vi "Event from DBL Ary.vi"(7 "Time Stamp":timestamp, 10 "Array":dbl[](array[numeric]), 11 "VI Refnum":refnum<vi>) -> (2 "Event Data":T1)   [LabVIEW 2023, in "Instruments.lvlib" / "Instruments.lvclass"]
uses:
  Library/Instruments.lvclass
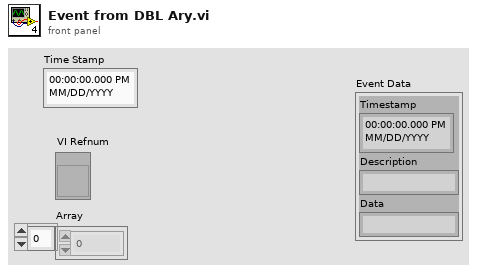
[diagram p1: front panel]
types:
  T1 = cluster{"Timestamp":timestamp, "Description":string, "Data":string}
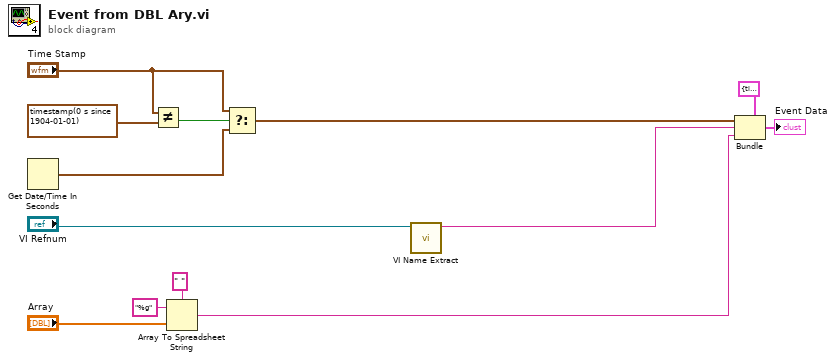
[diagram p0: block diagram]
diagram:
  n1 = Get Date/Time In Seconds() -> (seconds since 1Jan1904=w8:timestamp)
  n2 = Not Equal?(x="Time Stamp", y=timestamp(0 s since 1904-01-01) ("Time Stamp")) -> (x != y?=w10:bool)
  n3 = Array To Spreadsheet String(delimiter (Tab)=" ", array="Array", 3:"%g" ("format string")) -> (spreadsheet string=w5:string)
  n4 = Select(t="Time Stamp", s=w10, f=w8) -> (s? t:f=w7:timestamp)
  n5 = call "VI Name Extract.vi"("VI Refnum"="VI Refnum") -> ("Name"=w1:string)  [unwired: 10 in]
  n6 = Bundle(cluster=T1 {"Timestamp"=timestamp(0 s since 1904-01-01), "Description"="", "Data"=""}, "Timestamp"=w7, "Description"=w1, "Data"=w5) -> (→"Event Data":T1)
